vi "HFRR ADV v07.vi"() -> ()   [LabVIEW 2025] (continued)
            n790 = call "EDGE DETCTION.vi"("GAIN VALUE"=w877, "Image Path"=w876) -> ("error out"=w875:errorcluster, "return value"=w874:cluster{string, string, dbl, dbl, dbl})  [unwired: 8 in]
            n791 = Bundle By Name(cluster=T18 {"File Name"="", "Test Method"="", "Operator"="", "Fuel Description"="", "Date and time"=""} ("Main Ref"), "File Name"=w869) -> (w870:T18)
            n792 = call "duf file read.vi"("error in (no error)"=w875, "Main Ref"=w870) -> ("error out"=w873:errorcluster, "Main Ref 2"=w871:T18)  [unwired: 8 in]
            n793 = call "EDGE DETECTION REPORT.vi"("error in (no error)"=w873, "return value 2"=w874, "Main Ref"=w871) -> ()  [unwired: 8 in, 1 out]
          }
          frame #6 {
            n794 = property on="Auto Scar Check  2" class="Clust (strict)"("Visible"=FALSE) -> ()  [unwired: 2 in, 2 out]
          }
          frame #7 {
            n795 = call "CAMERA LIVE FEED FGV.vi"("Enum - Menu"=CAMERA_LIVE_FEED_ENUM."CAMERA MINIMIZE", "error in (no error)"=w884) -> ()  [unwired: 8 in, 2 out]
            n796 = local write "Main Dashboard Buttons"(T2."Home" ("Main Dashboard Buttons")) -> ()
            n797 = local write "Main Tab"(T3."HOME" ("Main Tab")) -> ()
          }
        }
      }
    }
    n798 = local read "Heater Button"() -> (w795:bool)
    n799 = case shown="True" w797 {
      selector: w797 -> [_ w1005]
      frame False {
      }
      frame True {
        n800 = Not(x=w1005) -> (.not. x?=w1003:bool)
        n801 = local write "Frequency"(w1003) -> ()
        n802 = local write "Tab Control 2"(T7."Frequency" ("Tab Control 2")) -> ()
      }
    }
    n803 = case shown="True" w796 {
      selector: w796 -> [_ w1002]
      frame False {
      }
      frame True {
        n804 = Not(x=w1002) -> (.not. x?=w1000:bool)
        n805 = local write "Air Temp vs Humidity"(w1000) -> ()
        n806 = local write "Tab Control 2"(T7."Air Temp vs Rh" ("Tab Control 2")) -> ()
      }
    }
    n807 = case shown="True" w798 {
      selector: w798 -> [_ w1008]
      frame False {
      }
      frame True {
        n808 = Not(x=w1008) -> (.not. x?=w1006:bool)
        n809 = local write "Sample Temperature"(w1006) -> ()
        n810 = local write "Tab Control 2"(T7."Sample Temperature" ("Tab Control 2")) -> ()
      }
    }
    n811 = case shown="\"Custom\"" w794 {
      frame "ASTM D6079", Default {
        w981 = "ASTM D6079 TEST CONDITIONS" ("Standard 2")
        n812 = local write "Standard 2"(w981) -> ()
        n813 = local write "Standard"(w981) -> ()
      }
      frame "ISO 12156" {
        w982 = "ISO 12156 TEST CONDITIONS" ("Standard 2")
        n814 = local write "Standard 2"(w982) -> ()
        n815 = local write "Standard"(w982) -> ()
      }
      frame "CEC F-096-A-06" {
        w983 = "CEC F-096-A-06 TEST CONDITIONS" ("Standard 2")
        n816 = local write "Standard 2"(w983) -> ()
        n817 = local write "Standard"(w983) -> ()
      }
      frame "Custom" {
        w984 = "CUSTOM TEST CONDITIONS" ("Standard 2")
        n818 = local write "Standard 2"(w984) -> ()
        n819 = local write "Standard"(w984) -> ()
      }
    }
    n820 = case shown="True" w795 {
      frame False {
        n821 = local write "Temperature On Command"(TRUE ("Temperature On Command")) -> ()
        n822 = case shown="True" "Temperature Off Command" {
          selector: "Temperature Off Command" -> [_ w988]
          frame False {
          }
          frame True {
            n823 = Not(x=w988) -> (.not. x?=w987:bool)
            n824 = local read "EVENT LOG"() -> (w991:string)
            n825 = local write "Temperature Off Command"(w987) -> ()
            n826 = call "Event Log.vi"("Content"="Heater Off", "EVENT LOG"=w991) -> ("EVENT LOG"=w990:string)  [unwired: 8 in, 1 out]
            n827 = local write "EVENT LOG"(w990) -> ()
          }
        }
      }
      frame True {
        n828 = local write "Temperature Off Command"(TRUE ("Temperature Off Command")) -> ()
        n829 = case shown="True" "Temperature On Command" {
          selector: "Temperature On Command" -> [_ w995]
          frame False {
          }
          frame True {
            n830 = Not(x=w995) -> (.not. x?=w994:bool)
            n831 = local write "Temperature On Command"(w994) -> ()
            n832 = disable-structure shown="Enabled" {
              disable-tunnel: "Heater On" -> [w997 _]
              frame Enabled {
                n833 = local read "EVENT LOG"() -> (w998:string)
                n834 = call "Event Log.vi"("Content"=w997, "EVENT LOG"=w998) -> ("EVENT LOG"=w999:string)  [unwired: 8 in, 1 out]
                n835 = local write "EVENT LOG"(w999) -> ()
              }
              frame Disabled {
              }
            }
          }
        }
      }
    }
    n836 = local read "Main Tab"() -> (w786:T3)
    n837 = case shown="\"Acquire\"" w786 {
      frame "HOME", Default {
        w830 = T15."Enabled" ("Disabled")
        n838 = property on="Imaging" class="Bool (strict)"("DisabledEnum"=w830) -> ()  [unwired: 2 in, 2 out]
        n839 = property on="Dashboard" class="Bool (strict)"("DisabledEnum"=w830) -> ()  [unwired: 2 in, 2 out]
        n840 = property on="About" class="Bool (strict)"("DisabledEnum"=w830) -> ()  [unwired: 2 in, 2 out]
        n841 = property on="Test Setup" class="Bool (strict)"("DisabledEnum"=w830) -> ()  [unwired: 2 in, 2 out]
        n842 = property on="Analysis" class="Bool (strict)"("DisabledEnum"=w830) -> ()  [unwired: 2 in, 2 out]
        n843 = property on="Main Dashboard Buttons" class="RadioBtnsControl (strict)"("DisabledEnum"=w830) -> ()  [unwired: 2 in, 2 out]
        n844 = property on="Home" class="Bool (strict)"("DisabledEnum"=w830) -> ()  [unwired: 2 in, 2 out]
        n845 = property on="Report" class="Bool (strict)"("DisabledEnum"=w830) -> ()  [unwired: 2 in, 2 out]
      }
      frame "Test Setup" {
        w831 = T15."Enabled" ("Disabled")
        n846 = property on="Dashboard" class="Bool (strict)"("DisabledEnum"=T15."Disabled" ("Disabled")) -> ()  [unwired: 2 in, 2 out]
        n847 = property on="Imaging" class="Bool (strict)"("DisabledEnum"=w831) -> ()  [unwired: 2 in, 2 out]
        n848 = property on="About" class="Bool (strict)"("DisabledEnum"=w831) -> ()  [unwired: 2 in, 2 out]
        n849 = property on="Test Setup" class="Bool (strict)"("DisabledEnum"=w831) -> ()  [unwired: 2 in, 2 out]
        n850 = property on="Analysis" class="Bool (strict)"("DisabledEnum"=w831) -> ()  [unwired: 2 in, 2 out]
        n851 = property on="Home" class="Bool (strict)"("DisabledEnum"=w831) -> ()  [unwired: 2 in, 2 out]
        n852 = property on="Report" class="Bool (strict)"("DisabledEnum"=w831) -> ()  [unwired: 2 in, 2 out]
      }
      frame "Acquire" {
        n853 = local read "RUN"() -> (w833:bool)
        n854 = case shown="False" w833 {
          tunnel: [T15."Enabled" ("Disabled") T15."Disabled" ("Disabled")] -> w836
          frame False {
          }
          frame True {
          }
        }
        n855 = property on="Test Setup" class="Bool (strict)"("DisabledEnum"=T15."Disabled" ("Disabled")) -> ()  [unwired: 2 in, 2 out]
        n856 = property on="About" class="Bool (strict)"("DisabledEnum"=T15."Enabled" ("Disabled")) -> ()  [unwired: 2 in, 2 out]
        n857 = property on="Imaging" class="Bool (strict)"("DisabledEnum"=w836) -> ()  [unwired: 2 in, 2 out]
        n858 = property on="Dashboard" class="Bool (strict)"("DisabledEnum"=w836) -> ()  [unwired: 2 in, 2 out]
        n859 = property on="Analysis" class="Bool (strict)"("DisabledEnum"=w836) -> ()  [unwired: 2 in, 2 out]
        n860 = property on="Home" class="Bool (strict)"("DisabledEnum"=w836) -> ()  [unwired: 2 in, 2 out]
        n861 = property on="Report" class="Bool (strict)"("DisabledEnum"=w836) -> ()  [unwired: 2 in, 2 out]
      }
    }
    n862 = local read "Quit"() -> (w814:bool)
    "Single" <- "Single - Graph"
  }
  n863 = disable-structure shown="Disabled" {
    disable-tunnel: [w1073 _] -> w29
    disable-tunnel: _ -> [w1072 _]
    frame Disabled {
      n864 = while {
        tunnel: w1072 -> [_]
        tunnel: [w1074] -> w1073
        tunnel: [w1075] -> _
        i -> [w1075]
        stop <- w1074 stop-if-true
        w1091 = u16 10 items=["1.0"=10, "1.5"=15, "2.0"=20] ("stop bits (10: 1 bit)")
        n865 = Wait (ms)(milliseconds to wait=u32 10) -> ()  [unwired: 1 out]
        n866 = call-poly "VISA Configure Serial Port"("VISA resource name"=refnum<visa-resource-name> "ASRL1::INSTR" ("COM PORT"), "timeout (10sec)"=u32 10, "baud rate (9600)"=u32 57600, "data bits (8)"=u16 8, "stop bits (10: 1 bit)"=w1091) -> ("VISA resource name out"=w1077:refnum<visa-resource-name>, "error out"=w1086:errorcluster)  [unwired: 9 in]
        n867 = VISA Read(VISA resource name=w1077, byte count=u32 2 ("byte count (0)")) -> (read buffer=w1085:string)  [unwired: 1 in, 3 out]
        n868 = String Subset(string=w1085, offset (0)=0, length (rest)=2 ("length (rest)")) -> (substring=w1084:string)
        n869 = Match Pattern(string=w1084, regular expression="<>") -> (offset past match=w1081:i32)  [unwired: 1 in, 3 out]
        n870 = Greater Or Equal?(x=w1081, y=0) -> (x >= y?=w1076:bool)
        n871 = case shown="True" w1076 {
          tunnel: w1077 -> [_ w1095]
          tunnel: w1086 -> [_ w1094]
          frame False {
          }
          frame True {
            n872 = VISA Read(VISA resource name=w1095, byte count=u32 32 ("byte count (0)"), error in (no error)=w1094) -> (read buffer=w1093:string)  [unwired: 3 out]
            n873 = String Subset(string=w1093, offset (0)=0, length (rest)=8 ("length (rest)")) -> (substring=w1097:string)
            n874 = String Subset(string=w1093, offset (0)=8, length (rest)=8 ("length (rest)")) -> (substring=w1098:string)
            n875 = Decimal String To Number(string=w1098) -> (number=w1105:i32)  [unwired: 2 in, 1 out]
            n876 = Decimal String To Number(string=w1097) -> (number=w1101:i32)  [unwired: 2 in, 1 out]
            n877 = Divide(x=w1105, y=10000) -> ()  [unwired: 1 out]
            n878 = Divide(x=w1101, y=1000000) -> ()  [unwired: 1 out]
          }
        }
        n879 = local read "Quit"() -> (w1074:bool)
      }
    }
    frame Enabled {
    }
  }
  n880 = local write "Err Count"(0 ("Err Count")) -> ()
  n881 = local write "FRICVALZ"(0.0 ("FRICVALZ")) -> ()
  n882 = Tick Count (ms)() -> (millisecond timer value=w42:u32)
  n883 = while {
    shift-right: [w1124] -> w46
    shift-left: _ -> [w1113]
    shift-right: [w1123] -> w45
    shift-left: errorcluster {"status"=TRUE, "code"=0, "source"="Init"} ("error IO") -> [w1115]
    shift-right: [w1121] -> _
    shift-left: w42 -> [w1122]
    tunnel: [w1107] -> w33
    tunnel: [w1120] -> _
    i -> [w1120]
    stop <- w1107 stop-if-true
    n884 = local read "Com Port 1"() -> (w1114:refnum<visa-resource-name>)
    n885 = local read "Port 1a"() -> (w1116:bool)
    n886 = local read "Port 3"() -> (w1117:bool)
    n887 = Not Equal?(x=w1114, y=w1113) -> (x != y?=w1112:bool)
    n888 = Or(x=w1117, y=w1116) -> (x .or. y?=w1119:bool)
    n889 = Unbundle(w1115) -> ("status"=→"Port 3":bool)  [unwired: 2 out]
    n890 = flat-sequence {
      tunnel: [w1127] -> w1111
      tunnel: w1115 -> [w1127]
      frame #0 {
        n891 = Wait (ms)(milliseconds to wait=u32 200) -> ()  [unwired: 1 out]
      }
    }
    n892 = case shown="False" w1119 {
      frame False {
        w1129 = FALSE ("Visible")
        n893 = property on="Port 1a" class="Bool (strict)"("Visible"=w1129) -> ()  [unwired: 2 in, 2 out]
        n894 = property on="Port 3" class="Bool (strict)"("Visible"=w1129) -> ()  [unwired: 2 in, 2 out]
      }
      frame True {
        w1130 = TRUE ("Visible")
        n895 = property on="Port 1a" class="Bool (strict)"("Visible"=w1130) -> ()  [unwired: 2 in, 2 out]
        n896 = property on="Port 3" class="Bool (strict)"("Visible"=w1130) -> ()  [unwired: 2 in, 2 out]
      }
    }
    n897 = local read "Re-Initialise"() -> (w1108:bool)
    n898 = Or(x=w1112, y=w1108) -> (x .or. y?=w1109:bool)
    n899 = case shown="True" w1109 {
      tunnel: [w1125 errorcluster {"status"=TRUE, "code"=0, "source"="Init"} ("error out")] -> w1110
      tunnel: w1111 -> [w1125 _]
      frame False {
      }
      frame True {
      }
    }
    n900 = case shown="No Error" w1110 {
      selector: w1110 -> [w1131 w1457]
      tunnel: [w1136 w1462] -> w1124
      tunnel: [w1135 w1454] -> w1123
      tunnel: w1113 -> [w1134 w1460]
      tunnel: w1122 -> [w1133 w1459]
      tunnel: [w1132 w1459] -> w1121
      frame No Error {
        n901 = stacked-sequence {
          tunnel: [w1146 _ _ _ _ _] -> w1136
          tunnel: [w1145 _ _ _ _ _] -> w1135
          tunnel: w1134 -> [w1141 _ _ _ _ _]
          tunnel: w1131 -> [w1140 _ _ _ _ _]
          tunnel: w1133 -> [_ w1254 _ _ _ _]
          tunnel: [_ w1253 _ _ _ _] -> w1132
          tunnel: [_ w1225 _ _ _ _] -> _
          frame #0 {
            n902 = property class="Instr"(reference=w1141, error in=w1140) -> (reference out=w1143:refnum<visa-resource-name>, error out=w1144:errorcluster, "Serial Settings:Number of Bytes at Serial Port"=w1137:u32)
            "Sps 3" <- w1137
            "Port 1" <- w1137
            n903 = Greater?(x=w1137, y=u32 5) -> (0:w1139:bool)
            n904 = case shown="True" w1139 {
              tunnel: w1143 -> [w1148 w1169]
              tunnel: w1144 -> [w1147 w1170]
              tunnel: [w1147 w1172] -> w1145
              tunnel: [w1148 w1171] -> w1146
              frame False {
              }
              frame True {
                # "Out as Volts"
                n905 = local read "Residual Uno"() -> (w1163:string)
                n906 = while {
                  tunnel: [w1209] -> w1172
                  tunnel: [w1208] -> w1171
                  tunnel: w1170 -> [w1207]
                  tunnel: w1169 -> [w1206]
                  tunnel: [w1203] -> _
                  shift-right: [w1199] -> w1151
                  shift-left: w1163 -> [w1201]
                  i -> [w1203]
                  stop <- w1204 stop-if-true
                  n907 = property class="Instr"(reference=w1206, error in=w1207) -> (reference out=w1211:refnum<visa-resource-name>, error out=w1210:errorcluster, "Serial Settings:Number of Bytes at Serial Port"=w1202:u32)
                  n908 = VISA Read(VISA resource name=w1211, byte count=w1202, error in (no error)=w1210) -> (VISA resource name out=w1208:refnum<visa-resource-name>, read buffer=w1200:string, error out=w1209:errorcluster)  [unwired: 1 out]
                  n909 = Greater?(x=w1202, y=u32 30) -> (0:w1204:bool)
                  n910 = Concatenate Strings(w1201, w1200) -> (w1199:string)
                }
                "UnoRead" <- w1151
                n911 = while {
                  shift-right: [w1185] -> w1162
                  shift-left: w1151 -> [w1191]
                  tunnel: [w1184] -> w1158 mode=indexing
                  tunnel: [w1186] -> _
                  i -> [w1186]
                  stop <- w1188 stop-if-true
                  n912 = Match Pattern(string=w1191, regular expression="*") -> (after substring=w1189:string)  [unwired: 1 in, 3 out]
                  n913 = Match Pattern(string=w1189, regular expression="&") -> (before substring=w1184:string, after substring=w1185:string, offset past match=w1187:i32)  [unwired: 1 in, 1 out]
                  n914 = Less Than 0?(x=w1187) -> (x < 0?=w1188:bool)
                }
                n915 = local write "Residual Uno"(w1162) -> ()
                n916 = Array Size(array=w1158) -> (size(s)=w1159:i32)
                n917 = Decrement(x=w1159) -> (x-1=w1161:i32)
                n918 = Delete From Array(array=w1158, length=1, index=w1161) -> (array with subset deleted=w1156:string[])  [unwired: 1 out]
                n919 = Array Size(array=w1156) -> (size(s)=w1155:i32)
                n920 = Decrement(x=w1155) -> (x-1=w1154:i32)
                n921 = while {
                  tunnel: [w1183] -> w1167 mode=indexing
                  tunnel: [w1182] -> w1166 mode=indexing
                  tunnel: w1156 -> [w1176] mode=indexing
                  tunnel: w1154 -> [w1175]
                  tunnel: [w1173] -> _
                  i -> [w1173]
                  stop <- w1174 stop-if-true
                  w1177 = 0 ("length (rest)")
                  w1179 = ";" ("regular expression")
                  n922 = Less Or Equal?(x=w1175, y=w1173) -> (x <= y?=w1174:bool)
                  n923 = Match Pattern(string=w1176, regular expression=w1179) -> (before substring=w1181:string, after substring=w1180:string)  [unwired: 1 in, 2 out]
                  n924 = Decimal String To Number(string=w1181, default (0L)=w1177) -> (number=w1183:i32)  [unwired: 1 in, 1 out]
                  n925 = Match Pattern(string=w1180, regular expression=w1179) -> (before substring=w1178:string)  [unwired: 1 in, 3 out]
                  n926 = Decimal String To Number(string=w1178, default (0L)=w1177) -> (number=w1182:i32)  [unwired: 1 in, 1 out]
                }
                n927 = case shown="0, Default" "ADC Res" {
                  tunnel: [w1194 w1196] -> w1150
                  frame 0, Default {
                    n928 = Divide(x=65535 ("length (rest)"), y=2 ("length (rest)")) -> (x/y=w1194:dbl)
                  }
                  frame 1 {
                    n929 = Divide(x=16777216 ("length (rest)"), y=2 ("length (rest)")) -> (x/y=w1196:dbl)
                  }
                }
                n930 = Bundle(w1167, w1166) -> (w1157:cluster{i32[], i32[]})  [unwired: 1 in]
                n931 = Divide(x=w1157, y=w1150) -> (x/y=w1168:cluster{dbl[], dbl[]})
                n932 = Multiply(x=w1168, y=sgl 5.03 ("Numeric")) -> (x*y=w1165:cluster{dbl[], dbl[]})
                n933 = Unbundle(w1165) -> (→"Ch1":dbl[], →"Ch0":dbl[])
              }
            }
            n934 = Not(x=w1139) -> (.not. x?=→"Port 1a":bool)
          }
          frame #1 {
            n935 = local read "zOff 2"() -> (w1246:dbl)
            n936 = local read "Ch1"() -> (w1236:dbl[])
            n937 = case shown="True" "Zero 2" {
              tunnel: w1236 -> [_ w1266]
              frame False {
              }
              frame True {
                n938 = call-poly <vilib>:"Mean.vi"("X"=w1266) -> ("mean"=→"zOff 2":dbl)  [unwired: 1 out]
                n939 = local write "Zero 2"(FALSE ("Zero")) -> ()
              }
            }
            n940 = Subtract(x=w1236, y=w1246) -> (x-y=w1242:dbl[])
            n941 = call-poly <vilib>:"Mean.vi"("X"=w1236) -> ("mean"=w1237:dbl)  [unwired: 1 out]
            "Slide 3" <- w1237
            n942 = Multiply(x=w1242, y=1.0 ("PG Oth")) -> (x*y=w1228:dbl[])
            n943 = local read "FF buffer"() -> (w1233:dbl[])
            n944 = Divide(x=w1228, y=1) -> (x/y=w1227:dbl[])
            "Fric Val" <- w1227
            n945 = call <vilib>:"Mean PtByPt.vi"("x"=w1237, "sample length"=10, "initialize"="Reset 2") -> ("mean"=→"Mean Pos Fil 2":dbl)  [unwired: 1 in, 1 out]
            n946 = Array Size(array=w1233) -> (size(s)=w1235:i32)
            n947 = call-poly <vilib>:"Mean.vi"("X"=w1227) -> ("mean"=w1241:dbl)  [unwired: 1 out]
            n948 = Insert Into Array(array=w1233, index=w1235, new element=w1227) -> (w1230:dbl[])
            n949 = Array Size(array=w1230) -> (size(s)=w1229:i32)
            n950 = case shown="True" "DC corr 2" {
              tunnel: w1227 -> [w1269 w1272]
              tunnel: [w1269 w1271] -> w1234
              tunnel: w1241 -> [_ w1270]
              frame False {
              }
              frame True {
                n951 = Subtract(x=w1272, y=w1270) -> (x-y=w1271:dbl[])
              }
            }
            n952 = Tick Count (ms)() -> (millisecond timer value=w1253:u32)
            n953 = Greater?(x=w1229, y=1000) -> (0:w1231:bool)
            n954 = Subtract(x=w1253, y=w1254) -> (x-y=w1252:u32)
            n955 = case shown="True" w1231 {
              tunnel: [w1259 w1262] -> w1218
              tunnel: w1230 -> [w1259 w1265]
              tunnel: w1229 -> [_ w1264]
              frame False {
              }
              frame True {
                n956 = Subtract(x=w1264, y=1000) -> (x-y=w1260:i32)
                n957 = Delete From Array(array=w1265, length=w1260, index=0) -> (array with subset deleted=w1262:dbl[])  [unwired: 1 out]
              }
            }
            n958 = Divide(x=w1252, y=u32 1000 ("x")) -> (x/y=w1250:dbl)
            n959 = Array Size(array=w1234) -> (size(s)=w1249:i32)
            n960 = Divide(x=w1249, y=w1250) -> (x/y=w1245:dbl)
            "Sps 2" <- w1245
            n961 = Reciprocal(x=w1245) -> (1/x=w1243:dbl)
            "dt" <- w1243
            n962 = local read "FRIC. FORCE :"() -> (w1215:dbl)
            n963 = local write "FF buffer"(w1218) -> ()
            n964 = Negate(x=w1218) -> (-x=w1217:dbl[])
            n965 = call "Elapsed Time5"("Time Target (s)"="check time s", "Reset"="Reset 3") -> ("Time has Elapsed"=w1220:bool)  [unwired: 10 in, 7 out]
            n966 = Array Max & Min(array=w1217) -> (max value=w1225:dbl)  [unwired: 3 out]
            n967 = Bundle By Name("Y"=w1234, "dt"=w1243, "t0"=timestamp(0 s since 1904-01-01)) -> (w1213:waveform(dbl))  [unwired: 1 in]
            n968 = Multiply(x=w1215, y=21.1986) -> (x*y=w1214:dbl)
            n969 = Greater Or Equal?(x=w1225, y="Threshold value") -> (x >= y?=w1221:bool)
            n970 = Multiply(x=w1214, y=w1213) -> (x*y=→"FF_Wfm":waveform(dbl))
            n971 = And(x=w1221, y=w1220) -> (x .and. y?=w1219:bool)
            n972 = case shown="True" w1219 {
              frame False {
                n973 = local write "Reset 3"(FALSE ("Reset 3")) -> ()
              }
              frame True {
                n974 = local write "Reset 3"(TRUE ("Reset 3")) -> ()
                n975 = local write "save dpt"(TRUE ("save dpt")) -> ()
              }
            }
          }
          frame #2 {
            n976 = local read "FF buffer"() -> (w1279:dbl[])
            n977 = Array Max & Min(array=w1279) -> (max value=w1274:dbl, min value=w1275:dbl)  [unwired: 2 out]
            n978 = Subtract(x=w1274, y=w1275) -> (x-y=w1276:dbl)
            n979 = Multiply(x=1.0 ("y 2"), y="Threshold") -> ()  [unwired: 1 out]
            n980 = Greater?(x=w1276, y="Threshold") -> (0:w1273:bool)
            n981 = case shown="True" w1273 {
              tunnel: w1279 -> [_ w1286]
              tunnel: [_ w1284] -> _
              frame False {
              }
              frame True {
                w1285 = 1.0 ("y")
                n982 = Delete From Array(array=w1286, length=100, index=0) -> (deleted portion=w1291:dbl[])  [unwired: 1 out]
                n983 = call-poly <vilib>:"Mean.vi"("X"=w1291) -> ("mean"=w1290:dbl)  [unwired: 1 out]
                n984 = Subtract(x=w1286, y=w1290) -> (x-y=w1289:dbl[])
                n985 = Multiply(x=w1285, y=w1285) -> (x*y=w1287:dbl)
                n986 = Multiply(x=w1289, y=w1287) -> (x*y=w1288:dbl[])
                "FF cal val" <- w1288
                n987 = Array Size(array=w1288) -> (size(s)=w1282:i32)
                n988 = Array Max & Min(array=w1288) -> (max value=w1281:dbl, min value=w1280:dbl)  [unwired: 2 out]
                n989 = property on="FF Calibration g" class="WFGraph (strict)"("X Scale.Range:Minimum"=0.0 ("y"), "X Scale.Range:Maximum"=w1282, "Y Scale.Range:Minimum"=w1281, "Y Scale.Range:Maximum"=w1280) -> ()  [unwired: 2 in, 2 out]
                n990 = local read "FRIC. FORCE :"() -> (w1284:dbl)
              }
            }
          }
          frame #3 {
            # "5"
            n991 = local read "DISPLACEMENT :"() -> (w1379:dbl)
            n992 = Multiply(x=w1379, y=1.0) -> (x*y=w1296:dbl)
            n993 = local read "zOff 3"() -> (w1382:dbl)
            n994 = local read "Ch0"() -> (w1309:dbl[])
            n995 = case shown="True" "Zero 3" {
              tunnel: w1309 -> [_ w1397]
              frame False {
              }
              frame True {
                n996 = call-poly <vilib>:"Mean.vi"("X"=w1397) -> ("mean"=→"zOff 3":dbl)  [unwired: 1 out]
                n997 = local write "Zero 3"(FALSE ("Zero")) -> ()
              }
            }
            n998 = Add(x=w1309, y="Offset") -> (x+y=w1308:dbl[])
            n999 = Multiply(x=w1296, y="DISPLACEMENT : 2") -> (x*y=w1363:dbl)
            n1000 = Subtract(x=w1309, y=w1382) -> (x-y=w1366:dbl[])
            n1001 = Multiply(x=w1366, y=w1363) -> (x*y=w1365:dbl[])
            n1002 = Multiply(x=w1366, y=w1296) -> (x*y=w1378:dbl[])
            "ABS DP" <- w1378
            n1003 = local read "Standard Slip Gauge (mm)"() -> (w1364:dbl)
            n1004 = call-poly <vilib>:"Mean.vi"("X"=w1365) -> ("mean"=w1295:dbl)  [unwired: 1 out]
            "Disp (mm)" <- w1295
            "software msrnt" <- w1295
            n1005 = Multiply(x=w1308, y="Gain") -> (x*y=w1303:dbl[])
            "Voltage LVDT Acq" <- w1303
            "gLVDTraw" <- w1303
            n1006 = call-poly <vilib>:"Mean.vi"("X"=w1378) -> ("mean"=w1368:dbl)  [unwired: 1 out]
            n1007 = case shown="True" "DC correction" {
              tunnel: w1378 -> [w1400 w1403]
              tunnel: [w1400 w1402] -> w1315
              tunnel: w1368 -> [_ w1401]
              frame False {
              }
              frame True {
                n1008 = Subtract(x=w1403, y=w1401) -> (x-y=w1402:dbl[])
              }
            }
            n1009 = Divide(x=w1295, y=w1364) -> (x/y=w1362:dbl)
            n1010 = call-poly <vilib>:"Mean.vi"("X"=w1303) -> ("mean"=w1302:dbl)  [unwired: 1 out]
            n1011 = Array Max & Min(array=w1303) -> (max value=w1307:dbl, min value=w1306:dbl)  [unwired: 2 out]
            n1012 = Multiply(x=w1362, y=w1363) -> (x*y=→"DISPLACEMENT : 3":dbl)
            n1013 = Subtract(x=w1307, y=w1306) -> (x-y=→"Pk-Pk":dbl)
            n1014 = local read "dt"() -> (w1381:dbl)
            n1015 = Threshold 1D Array(2:0.0 ("threshold y"), 3:w1315) -> (0:w1332:dbl)  [unwired: 1 in]
            n1016 = Bundle By Name("Y"=w1315, "dt"=w1381, "t0"=timestamp(0 s since 1904-01-01)) -> (w1370:waveform(dbl))  [unwired: 1 in]
            n1017 = local read "FF_Wfm"() -> (w1369:waveform(dbl))
            n1018 = Equal To 0?(x=w1332) -> (x = 0?=w1333:bool)
            n1019 = case shown="True" w1333 {
              tunnel: w1315 -> [_ w1391]
              tunnel: [w1387 w1388] -> w1328
              tunnel: w1332 -> [w1387 _]
              frame False {
              }
              frame True {
                n1020 = Threshold 1D Array(1:20 ("start index (0)"), 2:0.0 ("threshold y"), 3:w1391) -> (0:w1388:dbl)
              }
            }
            n1021 = call-poly <vilib>:"Extract Single Tone Information.vi"("time signal in"=w1370) -> ("detected amplitude"=w1304:dbl, "detected frequency"=→"Freq":dbl)  [unwired: 5 in, 4 out]
            n1022 = Build Array(w1370, w1369) -> (w1351:waveform(dbl)[])
            "Waveform Graph 2" <- w1351
            n1023 = Subtract(x=w1302, y="LvdtOff") -> (x-y=w1301:dbl)
            n1024 = Subtract(x=w1301, y=w1304) -> (x-y=w1313:dbl)
            n1025 = Add(x=w1304, y=w1301) -> (x+y=w1312:dbl)
            n1026 = Index Array(array=w1351) -> (element #1=w1352:waveform(dbl), element #2=w1354:waveform(dbl))  [unwired: 2 in]
            n1027 = Multiply(x=w1304, y=2.0) -> (x*y=w1371:dbl)
            "Stroke" <- w1371
            "Mean(RAW) Stroke" <- w1371
            n1028 = Bundle(w1301, w1313, w1312) -> (→"Slide 8":cluster{dbl, dbl, dbl})  [unwired: 1 in]
            n1029 = Unbundle By Name(w1352) -> ("Y"=w1325:dbl[])
            n1030 = Split 1D Array(array=w1315, index=w1328) -> (second subarray=w1329:dbl[])  [unwired: 1 out]
            n1031 = In Range and Coerce(upper limit=1.5, x=w1371, lower limit=0.5) -> (In Range?=w1375:bool)  [unwired: 1 out]
            n1032 = Split 1D Array(array=w1325, index="Window") -> (second subarray=w1343:dbl[])  [unwired: 1 out]
            n1033 = Unbundle By Name(w1354) -> ("Y"=w1326:dbl[])
            n1034 = Threshold 1D Array(1:180 ("start index (0)"), 2:0.0 ("threshold y"), 3:w1329) -> (0:w1327:dbl)
            n1035 = local read "Test \nStatus"() -> (w1372:bool)
            n1036 = Split 1D Array(array=w1326, index=w1328) -> (second subarray=w1323:dbl[])  [unwired: 1 out]
            n1037 = Not(x=w1375) -> (.not. x?=w1374:bool)
            n1038 = call-poly <vilib>:"RMS.vi"("X"=w1343) -> ("rms value"=w1299:dbl)  [unwired: 1 out]
            "Current (A)" <- w1299
            n1039 = Array Max & Min(array=w1343) -> (max value=w1357:dbl, min value=w1358:dbl)  [unwired: 2 out]
            n1040 = Array Max & Min(array=w1326) -> (max value=w1355:dbl, min value=w1356:dbl)  [unwired: 2 out]
            n1041 = Subtract(x=w1357, y=w1358) -> (x-y=w1359:dbl)
            n1042 = Subtract(x=w1355, y=w1356) -> (x-y=w1360:dbl)
            n1043 = And(x=w1374, y=w1372) -> (x .and. y?=w1373:bool)
            n1044 = Split 1D Array(array=w1329, index=w1327) -> (first subarray=w1322:dbl[])  [unwired: 1 out]
            n1045 = Split 1D Array(array=w1323, index=w1327) -> (first subarray=w1320:dbl[])  [unwired: 1 out]
            n1046 = case shown="True" w1373 {
              tunnel: [i32[] [] w1393] -> _
              frame False {
              }
              frame True {
                n1047 = local read "UnoRead"() -> (w1395:string)
                n1048 = local read "Array"() -> (w1396:string[])
                n1049 = Build Array (concatenate)(w1396, w1395) -> (w1394:string[])
                "Array" <- w1394
                n1050 = String Length(string=w1394) -> (length=w1393:i32[])
              }
            }
            n1051 = local read "G_val"() -> (w1345:dbl)
            n1052 = Divide(x=w1360, y=w1359) -> (x/y=w1348:dbl)
            n1053 = call-poly <vilib>:"RMS.vi"("X"=w1320) -> ("rms value"=w1344:dbl)  [unwired: 1 out]
            n1054 = call-poly <vilib>:"Hanning Window.vi"("X"=w1322) -> ("Windowed X"=w1321:dbl[])  [unwired: 1 out]
            n1055 = call-poly <vilib>:"Hanning Window.vi"("X"=w1320) -> ("Windowed X"=w1319:dbl[])  [unwired: 1 out]
            n1056 = local read "Constant (G)"() -> (w1337:dbl)
            n1057 = Divide(x=w1344, y=w1299) -> (x/y=w1338:dbl)
            n1058 = Build Array(w1321, w1319) -> (→"Waveform Graph 4":dbl[][])
            n1059 = Multiply(x=w1348, y=0.2) -> (x*y=w1350:dbl)
            n1060 = Multiply(x=0.8 ("y"), y=w1345) -> (x*y=w1349:dbl)
            n1061 = Add(x=w1350, y=w1349) -> (x+y=w1317:dbl)
            n1062 = Multiply(x=w1338, y=0.2) -> (x*y=w1339:dbl)
            n1063 = Multiply(x=0.8 ("y"), y=w1337) -> (x*y=w1340:dbl)
            n1064 = Add(x=w1339, y=w1340) -> (x+y=w1336:dbl)
            "Constant (G)" <- w1336
            n1065 = Not A Number/Path/Refnum?(number/path/refnum=w1317) -> (NaN/Path/Refnum?=w1316:bool)
            n1066 = Select(t=0.0, s=w1316, f=w1317) -> (s? t:f=w1297:dbl)
            "G_val" <- w1297
            n1067 = Multiply(x=w1299, y=w1297) -> (x*y=→"Friction Force (N)":dbl)
            n1068 = Bundle(w1336, "t"=w1297) -> (→"pk-pk":cluster{dbl, "t":dbl})  [unwired: 1 in]
          }
          frame #4 {
            # "C:\\WinDucom\\data\\"
            # "?C:\\LAB-IQ-NXT\\data"
            n1069 = case shown="True" "save dpt" {
              frame False {
              }
              frame True {
                n1070 = local write "save dpt"(FALSE ("Hold 3")) -> ()
                n1071 = local read "file count"() -> (w1407:i32)
                n1072 = Number To Decimal String(number=w1407) -> (decimal integer string=w1413:string)  [unwired: 1 in]
                n1073 = Add(x=1, y=w1407) -> (x+y=w1408:i32)
                n1074 = local write "file count"(w1408) -> ()
                n1075 = local read "FILE 2"() -> (w1412:string)
                n1076 = Concatenate Strings(w1412, w1413) -> (w1405:string)
                n1077 = Concatenate Strings("C:\\LAB-IQ\\data" ("Substring"), w1405) -> (w1420:string)
                n1078 = local read "FF buffer"() -> (w1415:dbl[])
                n1079 = local read "ABS DP"() -> (w1414:dbl[])
                n1080 = Concatenate Strings(w1420, ".dpf" ("Substring")) -> (w1418:string)
                n1081 = Build Array(w1415, w1414) -> (w1410:dbl[][])
                n1082 = Concatenate Strings("FF ( V ); DP( mincron ) " ("character string"), "\r") -> (w1424:string)
                n1083 = String To Path(string=w1418) -> (path=w1416:path)
                n1084 = Transpose 2D Array(2D array=w1410) -> (transposed array=w1409:dbl[][])
                n1085 = call <vilib>:"Write Characters To File.vi"("append to file? (new file:F)"=FALSE, "character string"=w1424, "file path (dialog if empty)"=w1416) -> ("new file path (Not A Path if cancelled)"=w1421:path)  [unwired: 2 in]
                n1086 = Array To Spreadsheet String(delimiter (Tab)=";", array=w1409, 3:"" ("format string")) -> (spreadsheet string=w1411:string)
                "String 9" <- w1411
                n1087 = call <vilib>:"Write Characters To File.vi"("append to file? (new file:F)"=TRUE, "character string"=w1411, "file path (dialog if empty)"=w1421) -> ()  [unwired: 2 in, 1 out]
              }
            }
          }
          frame #5 {
            n1088 = case shown="True" "Hold 4" {
              frame False {
              }
              frame True {
                n1089 = File Dialog(6:"*.dpf" ("pattern"), 11:path "C:/LAB-IQ" ("start path")) -> (0:w1431:errorcluster, 3:w1446:path)  [unwired: 5 in, 2 out]
                n1090 = Unbundle(w1431) -> ()  [unwired: 3 out]
                n1091 = call <vilib>:"Read Characters From File.vi"("file path (dialog if empty)"=w1446) -> ("character string"=w1436:string)  [unwired: 5 in, 3 out]
                n1092 = Spreadsheet String To Array(delimiter (Tab)=";", format string="%S", spreadsheet string=w1436, array type (2D Dbl)=string[][] []) -> (array=w1440:string[][])
                n1093 = for {
                  tunnel: w1440 -> [w1450] mode=indexing
                  tunnel: [w1449] -> w1441 mode=indexing
                  n1094 = for {
                    tunnel: w1450 -> [w1452] mode=indexing
                    tunnel: [w1451] -> w1449 mode=indexing
                    n1095 = call <vilib>:"Trim Whitespace.vi"("string"=w1452) -> ("trimmed string"=w1451:string)  [unwired: 1 in]
                  }
                }
                n1096 = Fract/Exp String To Number(string=w1441) -> (number=w1443:dbl[][])  [unwired: 3 in, 1 out]
                n1097 = Array Subset(array=w1443, index (row)=1 ("index (col)")) -> (w1445:dbl[][])  [unwired: 3 in]
                n1098 = Index Array(array=w1445, index (col) #1=0 ("disabled index (col)"), index (col) #2=1 ("disabled index (col)")) -> (element #1=w1434:dbl[], element #2=w1433:dbl[])  [unwired: 2 in]
                n1099 = Build Array(w1434, w1433) -> (→"Waveform Graph":dbl[][])
              }
            }
          }
        }
      }
      frame Error {
        w1468 = u16 0 items=["None", "XON/XOFF", "RTS/CTS", "XON/XOFF & RTS/CTS", "DTR/DSR", "XON/XOFF & DTR/DSR"] ("flow control (0:none)  2")
        w1466 = u16 10 items=["1.0"=10, "1.5"=15, "2.0"=20] ("stop bits 2")
        w1464 = u16 0 items=["None", "Odd", "Even", "Mark", "Space"] ("parity 2")
        w1465 = u32 10000  # timeout (10sec)
        n1100 = VISA Close(VISA resource name=w1460, error in (no error)=w1457) -> (error out=w1461:errorcluster)
        n1101 = local write "Sps 3"(0.0 ("Sps 4")) -> ()
        n1102 = call <vilib>:"Clear Errors.vi"("error in (no error)"=w1461) -> ("error out"=w1458:errorcluster)  [unwired: 5 in, 1 out]
        n1103 = local read "Com Port 1"() -> (w1453:refnum<visa-resource-name>)
        n1104 = call-poly "VISA Configure Serial Port"("VISA resource name"=w1453, "timeout (10sec)"=w1465, "baud rate (9600)"=u32 250000 ("baud rate  2"), "data bits (8)"=u16 8 ("data bits  2"), "parity (0:none)"=w1464, "error in (no error)"=w1458, "stop bits (10: 1 bit)"=w1466, "flow control (0:none)"=w1468) -> ("VISA resource name out"=w1469:refnum<visa-resource-name>, "error out"=w1470:errorcluster)  [unwired: 6 in]
        n1105 = flat-sequence {
          tunnel: w1469 -> [w1472]
          tunnel: w1470 -> [w1471]
          tunnel: [w1472] -> w1462
          tunnel: [w1471] -> w1454
          frame #0 {
            n1106 = Wait (ms)(milliseconds to wait=u32 50) -> ()  [unwired: 1 out]
          }
        }
        "Residual Uno" <- ""
        "Port 1 Error" <- w1454
      }
    }
    n1107 = local read "Quit"() -> (w1107:bool)
    "Error Uno" <- w1115
  }
  n1108 = while {
    shift-right: [w1489] -> w27
    shift-left: _ -> [w1480]
    shift-right: [w1488] -> w26
    shift-left: errorcluster {"status"=FALSE, "code"=0, "source"="Init"} ("error out") -> [w1482]
    tunnel: [w1474] -> w32
    tunnel: [w1487] -> _
    i -> [w1487]
    stop <- w1474 stop-if-true
    n1109 = local read "Com Port 2"() -> (w1481:refnum<visa-resource-name>)
    n1110 = local read "Port 2a"() -> (w1483:bool)
    n1111 = local read "Port 4"() -> (w1484:bool)
    n1112 = Not Equal?(x=w1481, y=w1480) -> (x != y?=w1479:bool)
    n1113 = Or(x=w1484, y=w1483) -> (x .or. y?=w1486:bool)
    n1114 = Unbundle(w1482) -> ("status"=→"Port 4":bool)  [unwired: 2 out]
    n1115 = flat-sequence {
      tunnel: w1482 -> [w1493]
      tunnel: [w1493] -> w1478
      frame #0 {
        n1116 = Wait (ms)(milliseconds to wait=u32 50) -> ()  [unwired: 1 out]
      }
    }
    n1117 = local read "Re-Initialise"() -> (w1475:bool)
    n1118 = case shown="True" w1486 {
      frame False {
        w1494 = FALSE ("Visible")
        n1119 = property on="Port 2a" class="Bool (strict)"("Visible"=w1494) -> ()  [unwired: 2 in, 2 out]
        n1120 = property on="Port 4" class="Bool (strict)"("Visible"=w1494) -> ()  [unwired: 2 in, 2 out]
      }
      frame True {
        w1495 = TRUE ("Visible")
        n1121 = property on="Port 2a" class="Bool (strict)"("Visible"=w1495) -> ()  [unwired: 2 in, 2 out]
        n1122 = property on="Port 4" class="Bool (strict)"("Visible"=w1495) -> ()  [unwired: 2 in, 2 out]
      }
    }
    n1123 = Or(x=w1479, y=w1475) -> (x .or. y?=w1476:bool)
    n1124 = case shown="True" w1476 {
      tunnel: [w1490 errorcluster {"status"=TRUE, "code"=0, "source"="Init"} ("error out")] -> w1477
      tunnel: w1478 -> [w1490 _]
      frame False {
      }
      frame True {
      }
    }
    n1125 = case shown="Error" w1477 {
      selector: w1477 -> [w1496 w1650]
      tunnel: [w1498 w1655] -> w1489
      tunnel: [w1497 w1648] -> w1488
      tunnel: w1480 -> [w1500 w1653]
      tunnel: [w1499 _] -> _
      frame No Error {
        n1126 = stacked-sequence {
          tunnel: w1500 -> [w1524 _]
          tunnel: w1496 -> [w1523 _]
          tunnel: [w1510 _] -> w1499
          tunnel: [w1509 _] -> w1498
          tunnel: [w1508 _] -> w1497
          frame #0 {
            n1127 = property class="Instr"(reference=w1524, error in=w1523) -> (reference out=w1507:refnum<visa-resource-name>, error out=w1522:errorcluster, "Serial Settings:Number of Bytes at Serial Port"=w1503:u32)
            "Port 2" <- w1503
            n1128 = Greater?(x=w1503, y=u32 23) -> (0:w1505:bool)
            n1129 = Not(x=w1505) -> ()  [unwired: 1 out]
            n1130 = case shown="True" w1505 {
              tunnel: w1507 -> [w1539 w1564]
              tunnel: w1522 -> [w1538 w1565]
              tunnel: [w1538 w1567] -> w1518
              tunnel: [w1539 w1566] -> w1519
              frame False {
              }
              frame True {
                # "Out as Volts"
                n1131 = local read "Residual Due"() -> (w1563:string)
                n1132 = while {
                  tunnel: [w1607] -> w1567
                  tunnel: [w1606] -> w1566
                  tunnel: w1565 -> [w1605]
                  tunnel: w1564 -> [w1604]
                  tunnel: [w1601] -> _
                  shift-right: [w1599] -> w1562
                  shift-left: w1563 -> [w1598]
                  i -> [w1601]
                  stop <- w1602 stop-if-true
                  n1133 = property class="Instr"(reference=w1604, error in=w1605) -> (reference out=w1609:refnum<visa-resource-name>, error out=w1608:errorcluster, "Serial Settings:Number of Bytes at Serial Port"=w1600:u32)
                  n1134 = VISA Read(VISA resource name=w1609, byte count=w1600, error in (no error)=w1608) -> (VISA resource name out=w1606:refnum<visa-resource-name>, read buffer=w1597:string, error out=w1607:errorcluster)  [unwired: 1 out]
                  n1135 = Greater?(x=w1600, y=u32 8) -> (0:w1602:bool)
                  n1136 = Concatenate Strings(w1598, w1597) -> (w1599:string)
                }
                n1137 = while {
                  shift-right: [w1590] -> w1546
                  shift-left: w1562 -> [w1595]
                  tunnel: [w1589] -> w1558 mode=indexing
                  tunnel: [w1588] -> _
                  i -> [w1588]
                  stop <- w1592 stop-if-true
                  n1138 = Match Pattern(string=w1595, regular expression="*") -> (after substring=w1593:string)  [unwired: 1 in, 3 out]
                  n1139 = Match Pattern(string=w1593, regular expression="&") -> (before substring=w1589:string, after substring=w1590:string, offset past match=w1591:i32)  [unwired: 1 in, 1 out]
                  n1140 = Less Than 0?(x=w1591) -> (x < 0?=w1592:bool)
                }
                n1141 = Array Size(array=w1558) -> (size(s)=w1561:i32)
                n1142 = local write "Residual Due"(w1546) -> ()
                n1143 = Decrement(x=w1561) -> (x-1=w1559:i32)
                n1144 = Delete From Array(array=w1558, length=1, index=w1559) -> (array with subset deleted=w1557:string[])  [unwired: 1 out]
                n1145 = Array Size(array=w1557) -> (size(s)=w1545:i32)
                n1146 = Decrement(x=w1545) -> (x-1=w1544:i32)
                n1147 = while {
                  tunnel: w1557 -> [w1576] mode=indexing
                  tunnel: w1544 -> [w1575]
                  tunnel: [w1573] -> w1552 mode=indexing
                  tunnel: [w1572] -> w1551 mode=indexing
                  tunnel: [w1571] -> w1550 mode=indexing
                  tunnel: [w1570] -> w1549 mode=indexing
                  tunnel: [w1569] -> w1547 mode=indexing
                  tunnel: [w1568] -> _
                  i -> [w1568]
                  stop <- w1574 stop-if-true
                  w1585 = u32 0 ("length (rest)")
                  w1584 = ";" ("regular expression")
                  n1148 = Less Or Equal?(x=w1575, y=w1568) -> (x <= y?=w1574:bool)
                  n1149 = Match Pattern(string=w1576, regular expression=w1584) -> (before substring=w1577:string, after substring=w1578:string)  [unwired: 1 in, 2 out]
                  n1150 = Match Pattern(string=w1578, regular expression=w1584) -> (before substring=w1581:string, after substring=w1579:string)  [unwired: 1 in, 2 out]
                  n1151 = Decimal String To Number(string=w1577, default (0L)=w1585) -> (number=w1573:u32)  [unwired: 1 in, 1 out]
                  n1152 = Decimal String To Number(string=w1581, default (0L)=w1585) -> (number=w1572:u32)  [unwired: 1 in, 1 out]
                  n1153 = Match Pattern(string=w1579, regular expression=w1584) -> (before substring=w1582:string, after substring=w1580:string)  [unwired: 1 in, 2 out]
                  n1154 = Decimal String To Number(string=w1582, default (0L)=w1585) -> (number=w1571:u32)  [unwired: 1 in, 1 out]
                  n1155 = Match Pattern(string=w1580, regular expression=w1584) -> (before substring=w1583:string, after substring=w1587:string)  [unwired: 1 in, 2 out]
                  n1156 = Decimal String To Number(string=w1583, default (0L)=w1585) -> (number=w1570:u32)  [unwired: 1 in, 1 out]
                  n1157 = Decimal String To Number(string=w1587, default (0L)=u8 0 ("length (rest)")) -> (number=w1569:u8)  [unwired: 1 in, 1 out]
                }
                "Din" <- w1547
                n1158 = Bundle(w1552, w1551, w1550, w1549) -> (w1554:cluster{u32[], u32[], u32[], u32[]})  [unwired: 1 in]
                n1159 = Divide(x=w1554, y=4095 ("length (rest)")) -> (x/y=w1556:cluster{dbl[], dbl[], dbl[], dbl[]})
                n1160 = Multiply(x=w1556, y=sgl 3.32 ("Numeric")) -> (x*y=w1548:cluster{dbl[], dbl[], dbl[], dbl[]})
                n1161 = Unbundle(w1548) -> (→"ECR":dbl[], →"Rtemp":dbl[], →"Air temp":dbl[], →"Ch3 2":dbl[])
              }
            }
            n1162 = call "Elapsed Time10"("Time Target (s)"=2.0, "Reset"=w1505, "Auto Reset"=FALSE) -> ("Time has Elapsed"=→"Port 2a":bool)  [unwired: 9 in, 7 out]
            n1163 = local read "Due Com"() -> (w1511:string[])
            n1164 = Array Size(array=w1511) -> (size(s)=w1510:i32)
            n1165 = Delete From Array(array=w1511, length=1, index=0) -> (deleted portion=w1514:string[], array with subset deleted=w1515:string[])
            n1166 = local write "Due Com"(w1515) -> ()
            n1167 = Index Array(array=w1514, index=0) -> (element=w1512:string)
            n1168 = Not Equal?(x=w1512, y="") -> (x != y?=w1520:bool)
            n1169 = case shown="True" w1520 {
              tunnel: w1519 -> [w1526 w1531]
              tunnel: [w1526 w1535] -> w1509
              tunnel: w1518 -> [w1525 w1530]
              tunnel: [w1525 w1533] -> w1508
              tunnel: w1512 -> [_ w1529]
              tunnel: [_ w1532] -> _
              frame False {
                # "DATA  WRITE LOOP"
              }
              frame True {
                n1170 = Concatenate Strings(w1529, "\r\n") -> (w1528:string)
                n1171 = VISA Write(VISA resource name=w1531, write buffer=w1528, error in (no error)=w1530) -> (VISA resource name out=w1535:refnum<visa-resource-name>, return count=w1532:u32, error out=w1534:errorcluster)
                n1172 = flat-sequence {
                  tunnel: w1534 -> [w1536]
                  tunnel: [w1536] -> w1533
                  frame #0 {
                    n1173 = Wait (ms)(milliseconds to wait=u32 5) -> ()  [unwired: 1 out]
                  }
                }
              }
            }
          }
          frame #1 {
            w1618 = 10 ("y")
            w1623 = 10 ("y")
            n1174 = local read "Rtemp"() -> (w1611:dbl[])
            n1175 = local read "ecr buf"() -> (w1612:dbl[])
            n1176 = for {
              tunnel: w1611 -> [w1635] mode=indexing
              shift-right: [w1636] -> w1619
              shift-left: dbl[] [] ("temp buf 2") -> [w1637]
              n1177 = Build Array (concatenate)(w1637, w1635) -> (w1638:dbl[])
              n1178 = Equal To 0?(x=w1635) -> (x = 0?=w1639:bool)
              n1179 = Select(t=w1637, s=w1639, f=w1638) -> (s? t:f=w1636:dbl[])
            }
            n1180 = local read "ECR"() -> (w1610:dbl[])
            n1181 = Insert Into Array(array=w1610, index=0, new element=w1612) -> (w1616:dbl[])
            n1182 = local read "temp buf"() -> (w1620:dbl[])
            n1183 = Array Size(array=w1616) -> (size(s)=w1617:i32)
            n1184 = Greater?(x=w1617, y=w1618) -> (0:w1615:bool)
            n1185 = case shown="True" w1615 {
              tunnel: w1616 -> [w1628 w1634]
              tunnel: w1617 -> [_ w1632]
              tunnel: w1618 -> [_ w1631]
              tunnel: [w1628 w1629] -> w1613
              frame False {
              }
              frame True {
                n1186 = Subtract(x=w1632, y=w1631) -> (x-y=w1630:i32)
                n1187 = Delete From Array(array=w1634, length=w1630, index=0) -> (array with subset deleted=w1629:dbl[])  [unwired: 1 out]
              }
            }
            "ecr buf" <- w1613
            n1188 = Insert Into Array(array=w1619, index=0, new element=w1620) -> (w1625:dbl[])
            n1189 = Array Size(array=w1625) -> (size(s)=w1624:i32)
            n1190 = Greater?(x=w1624, y=w1623) -> (0:w1626:bool)
            n1191 = case shown="True" w1626 {
              tunnel: w1625 -> [w1640 w1646]
              tunnel: w1624 -> [_ w1644]
              tunnel: w1623 -> [_ w1643]
              tunnel: [w1640 w1641] -> w1622
              frame False {
              }
              frame True {
                n1192 = Subtract(x=w1644, y=w1643) -> (x-y=w1642:i32)
                n1193 = Delete From Array(array=w1646, length=w1642, index=0) -> (array with subset deleted=w1641:dbl[])  [unwired: 1 out]
              }
            }
            "temp buf" <- w1622
          }
        }
      }
      frame Error {
        w1661 = u16 0 items=["None", "XON/XOFF", "RTS/CTS", "XON/XOFF & RTS/CTS", "DTR/DSR", "XON/XOFF & DTR/DSR"] ("flow control (0:none)  2")
        w1659 = u16 10 items=["1.0"=10, "1.5"=15, "2.0"=20] ("stop bits 2")
        w1657 = u16 0 items=["None", "Odd", "Even", "Mark", "Space"] ("parity 2")
        w1658 = u32 10000  # timeout (10sec)
        n1194 = VISA Clear(VISA resource name=w1653, error in (no error)=w1650) -> (VISA resource name out=w1652:refnum<visa-resource-name>, error out=w1651:errorcluster)
        n1195 = VISA Close(VISA resource name=w1652, error in (no error)=w1651) -> (error out=w1654:errorcluster)
        n1196 = call <vilib>:"Clear Errors.vi"("error in (no error)"=w1654) -> ()  [unwired: 5 in, 2 out]
        n1197 = local read "Com Port 2"() -> (w1647:refnum<visa-resource-name>)
        "visa due" <- w1647
        n1198 = call-poly "VISA Configure Serial Port"("VISA resource name"=w1647, "timeout (10sec)"=w1658, "baud rate (9600)"=u32 250000 ("baud rate  2"), "data bits (8)"=u16 8 ("data bits  2"), "parity (0:none)"=w1657, "stop bits (10: 1 bit)"=w1659, "flow control (0:none)"=w1661) -> ("VISA resource name out"=w1662:refnum<visa-resource-name>, "error out"=w1663:errorcluster)  [unwired: 7 in]
        n1199 = flat-sequence {
          tunnel: w1662 -> [w1665]
          tunnel: w1663 -> [w1664]
          tunnel: [w1665] -> w1655
          tunnel: [w1664] -> w1648
          frame #0 {
            n1200 = Wait (ms)(milliseconds to wait=u32 50) -> ()  [unwired: 1 out]
          }
        }
        "Residual Due" <- ""
        "Port 2 Error" <- w1648
      }
    }
    n1201 = local read "Quit"() -> (w1474:bool)
    "Error Due" <- w1482
  }
  n1202 = property on="RUN" class="Bool (strict)"("Visible"=TRUE) -> ()  [unwired: 2 in, 2 out]
  n1203 = while {
    tunnel: [w1683] -> _
    tunnel: [w1667] -> w48
    i -> [w1683]
    stop <- w1667 stop-if-true
    n1204 = local read "conststatus"() -> (w1671:dbl)
    n1205 = local read "Main Tab"() -> (w1669:T3)
    n1206 = local read "EDIT"() -> (w1689:bool)
    n1207 = local read "Rate"() -> (w1688:dbl)
    n1208 = case shown="True" w1689 {
      tunnel: [FALSE TRUE] -> w1675
      frame False {
      }
      frame True {
      }
    }
    n1209 = property on="Time slide" class="Slide (strict)"("Scale.Range:Maximum"=2500.0) -> ()  [unwired: 2 in, 2 out]
    n1210 = Equal?(x=w1669, y=T19."About" ("Main Tab")) -> (x = y?=w1681:bool)
    n1211 = Equal?(x=w1671, y=0.0) -> (x = y?=w1672:bool)
    n1212 = Divide(x=1.0, y=w1688) -> (x/y=w1684:dbl)
    "Time 2" <- w1684
    n1213 = case shown="True" w1672 {
      frame False {
      }
      frame True {
        # "C:\\WinDucom\\calibrate WO 2391.dcf"
        n1214 = local write "Lan flag"(22) -> ()
        n1215 = local write "conststatus"(10.0 ("rpm value : 2")) -> ()
        n1216 = String To Path(string="C:\\LAB-IQ\\calibrate WO 2465.dcf") -> (path=w1695:path)
        n1217 = Open/Create/Replace File "Open File"(file path (use dialog)=w1695) -> (refnum out=w1693:refnum<file>)  [unwired: 5 in, 2 out]
        n1218 = for {
          N: 23 -> [_]
          tunnel: w1693 -> [w1704]
          i -> [w1698]
          (unwired) TRUE ("line mode (F)")
          n1219 = Read from Text File "Read File"(file (use dialog)=w1704) -> (text=w1703:string)  [unwired: 3 in, 3 out]
          n1220 = Match Pattern(string=w1703, regular expression="]") -> (after substring=w1701:string)  [unwired: 1 in, 3 out]
          n1221 = String Subset(string=w1703, offset (0)=5, length (rest)=10 ("length (rest)")) -> (substring=w1696:string)
          n1222 = Fract/Exp String To Number(string=w1696) -> (number=w1697:dbl)  [unwired: 3 in, 1 out]
          n1223 = Match Pattern(string=w1701, regular expression="-") -> (before substring=w1699:string)  [unwired: 1 in, 3 out]
          n1224 = case shown="7" w1698 {
            tunnel: w1697 -> [w1707 w1708 w1709 w1710 _ _ _ w1715 w1716 w1717 w1720 w1721 w1722 w1723 w1724 w1725 w1726 w1729 w1730 _ _ w1733 _ _]
            tunnel: w1699 -> [_ _ _ _ w1711 w1712 w1713 _ _ _ _ _ _ _ _ _ _ _ _ w1731 w1732 _ w1734 _]
            frame 0 {
              n1225 = local write "FRIC. FORCE :"(w1707) -> ()
            }
            frame 1 {
              n1226 = local write "TEMPERATURE :"(w1708) -> ()
            }
            frame 2 {
              n1227 = local write "HUMIDITY:"(w1709) -> ()
            }
            frame 3 {
              n1228 = local write "AIR TEMPERATURE :"(w1710) -> ()
            }
            frame 4 {
              n1229 = local write "Com Port 1"(w1711) -> ()
            }
            frame 5 {
              n1230 = local write "Com Port 2"(w1712) -> ()
              n1231 = local write "visa due"(w1712) -> ()
            }
            frame 6 {
              n1232 = String To Path(string=w1713) -> (path=w1714:path)
              n1233 = local write "File Path"(w1714) -> ()
              "String" <- w1713
            }
            frame 7 {
              n1234 = local write "DISPLACEMENT :"(w1715) -> ()
            }
            frame 8 {
              n1235 = local write "STROKE GAIN :"(w1716) -> ()
            }
            frame 9 {
              n1236 = local read "Stroke PID Gains"() -> (w1719:T9)
              n1237 = Bundle By Name(cluster=w1719, "Proportional Gain (Kc)"=w1717) -> (w1718:T9)
              n1238 = local write "Stroke PID Gains"(w1718) -> ()
            }
            frame 10 {
              n1239 = local write "Language Selection"(w1720) -> ()
            }
            frame 11 {
              n1240 = local write "CH-POWER +"(w1721) -> ()
            }
            frame 12 {
              n1241 = local write "CH-POWER -"(w1722) -> ()
            }
            frame 13 {
              n1242 = local write "CH-HEATER"(w1723) -> ()
            }
            frame 14 {
              n1243 = local write "CH-HUMIDITY WET"(w1724) -> ()
            }
            frame 15 {
              n1244 = local write "CH-HUMIDITY DRY"(w1725) -> ()
            }
            frame 16 {
              n1245 = local read "Stroke PID Gains"() -> (w1728:T9)
              n1246 = Bundle By Name(cluster=w1728, "Integral Time (Ti, min)"=w1726) -> (w1727:T9)
              n1247 = local write "Stroke PID Gains"(w1727) -> ()
            }
            frame 17 {
              n1248 = local write "AIR TEMP INTERCEPT:"(w1729) -> ()
            }
            frame 18 {
              n1249 = local write "TEMP INTERCEPT:"(w1730) -> ()
            }
            frame 19 {
              n1250 = local write "S.NO"(w1731) -> ()
            }
            frame 20 {
              n1251 = local write "Com Port 3"(w1732) -> ()
            }
            frame 21 {
              n1252 = local write "LvdtOff"(w1733) -> ()
            }
            frame 22 {
              n1253 = local write "Humidity :"(w1734) -> ()
            }
            frame 23, Default {
            }
          }
        }
      }
    }
    n1254 = Select(t=u32 2500 ("milliseconds to wait"), s=w1681, f=u32 500 ("milliseconds to wait")) -> (s? t:f=w1679:u32)
    n1255 = Multiply(x=w1684, y=w1679) -> (x*y=w1686:dbl)
